vi "RT_Angle_Of_Attack_in_DLR_Navigation_Reference_System_2_v2(SubVI).vi"(8 "i":i32, 9 "V_wind [m/s]":dbl[][](array[numeric]), 10 "Rotation":T1, 11 "output cluster 2":T3) -> (3 "output cluster":T2)   [LabVIEW 2017]
uses:
  <vilib>/Analysis/_algsub.llb/Vector Norm Type.ctl
  <vilib>/Analysis/_algsub.llb/Real Vector Norm.vi
  <vilib>/Analysis/coordinate.llb/Euler Rotation Order.ctl
  <vilib>/Analysis/NI_AALPro.lvlib
panel:
  out "Elevation [deg]":dbl
  out "Azimuth [deg]":dbl
  out "AoA_yaw (deg)":dbl
  out "AoA_pitch (deg)":dbl
  out "appended array":dbl[](array[numeric])
  out "Speed_quat":dbl[](array[numeric])
  out "pitch_stream (rad)":dbl
  out "yaw_stream (rad)":dbl
  out "AoA_yaw (rad)":dbl
  out "AoA_pitch (rad)":dbl
  out "VV":dbl[](array[numeric])
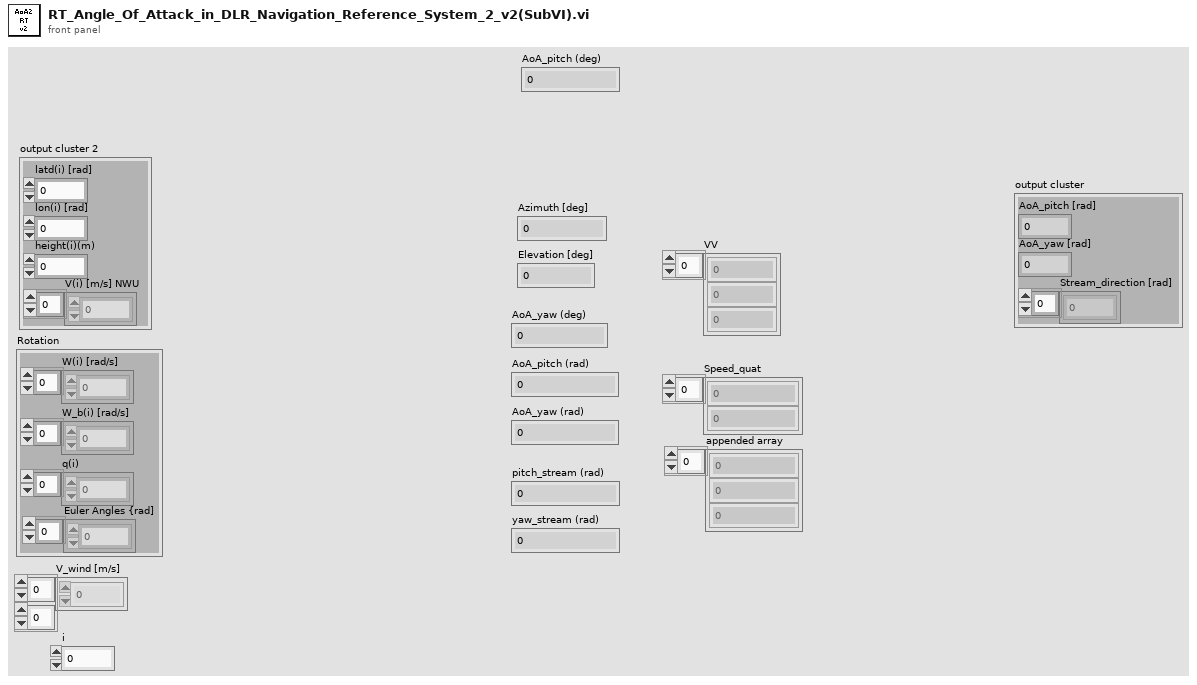
[diagram p1: front panel]
types:
  T1 = cluster{"W(i) [rad/s]":dbl[], "W_b(i) [rad/s]":dbl[], "q(i)":dbl[], "Euler Angles {rad]":dbl[]}
  T2 = cluster{"AoA_pitch [rad]":dbl, "AoA_yaw [rad]":dbl, "Stream_direction [rad]":dbl[]}
  T3 = cluster{"latd(i) [rad]":dbl, "lon(i) [rad]":dbl, "height(i)(m)":dbl, "V(i) [m/s] NWU":dbl[]}
  T4 = typedef "NI_AALPro.lvlib/Vector Norm Type.ctl" = u16
  T5 = typedef "NI_AALPro.lvlib/Euler Rotation Order.ctl" = u16
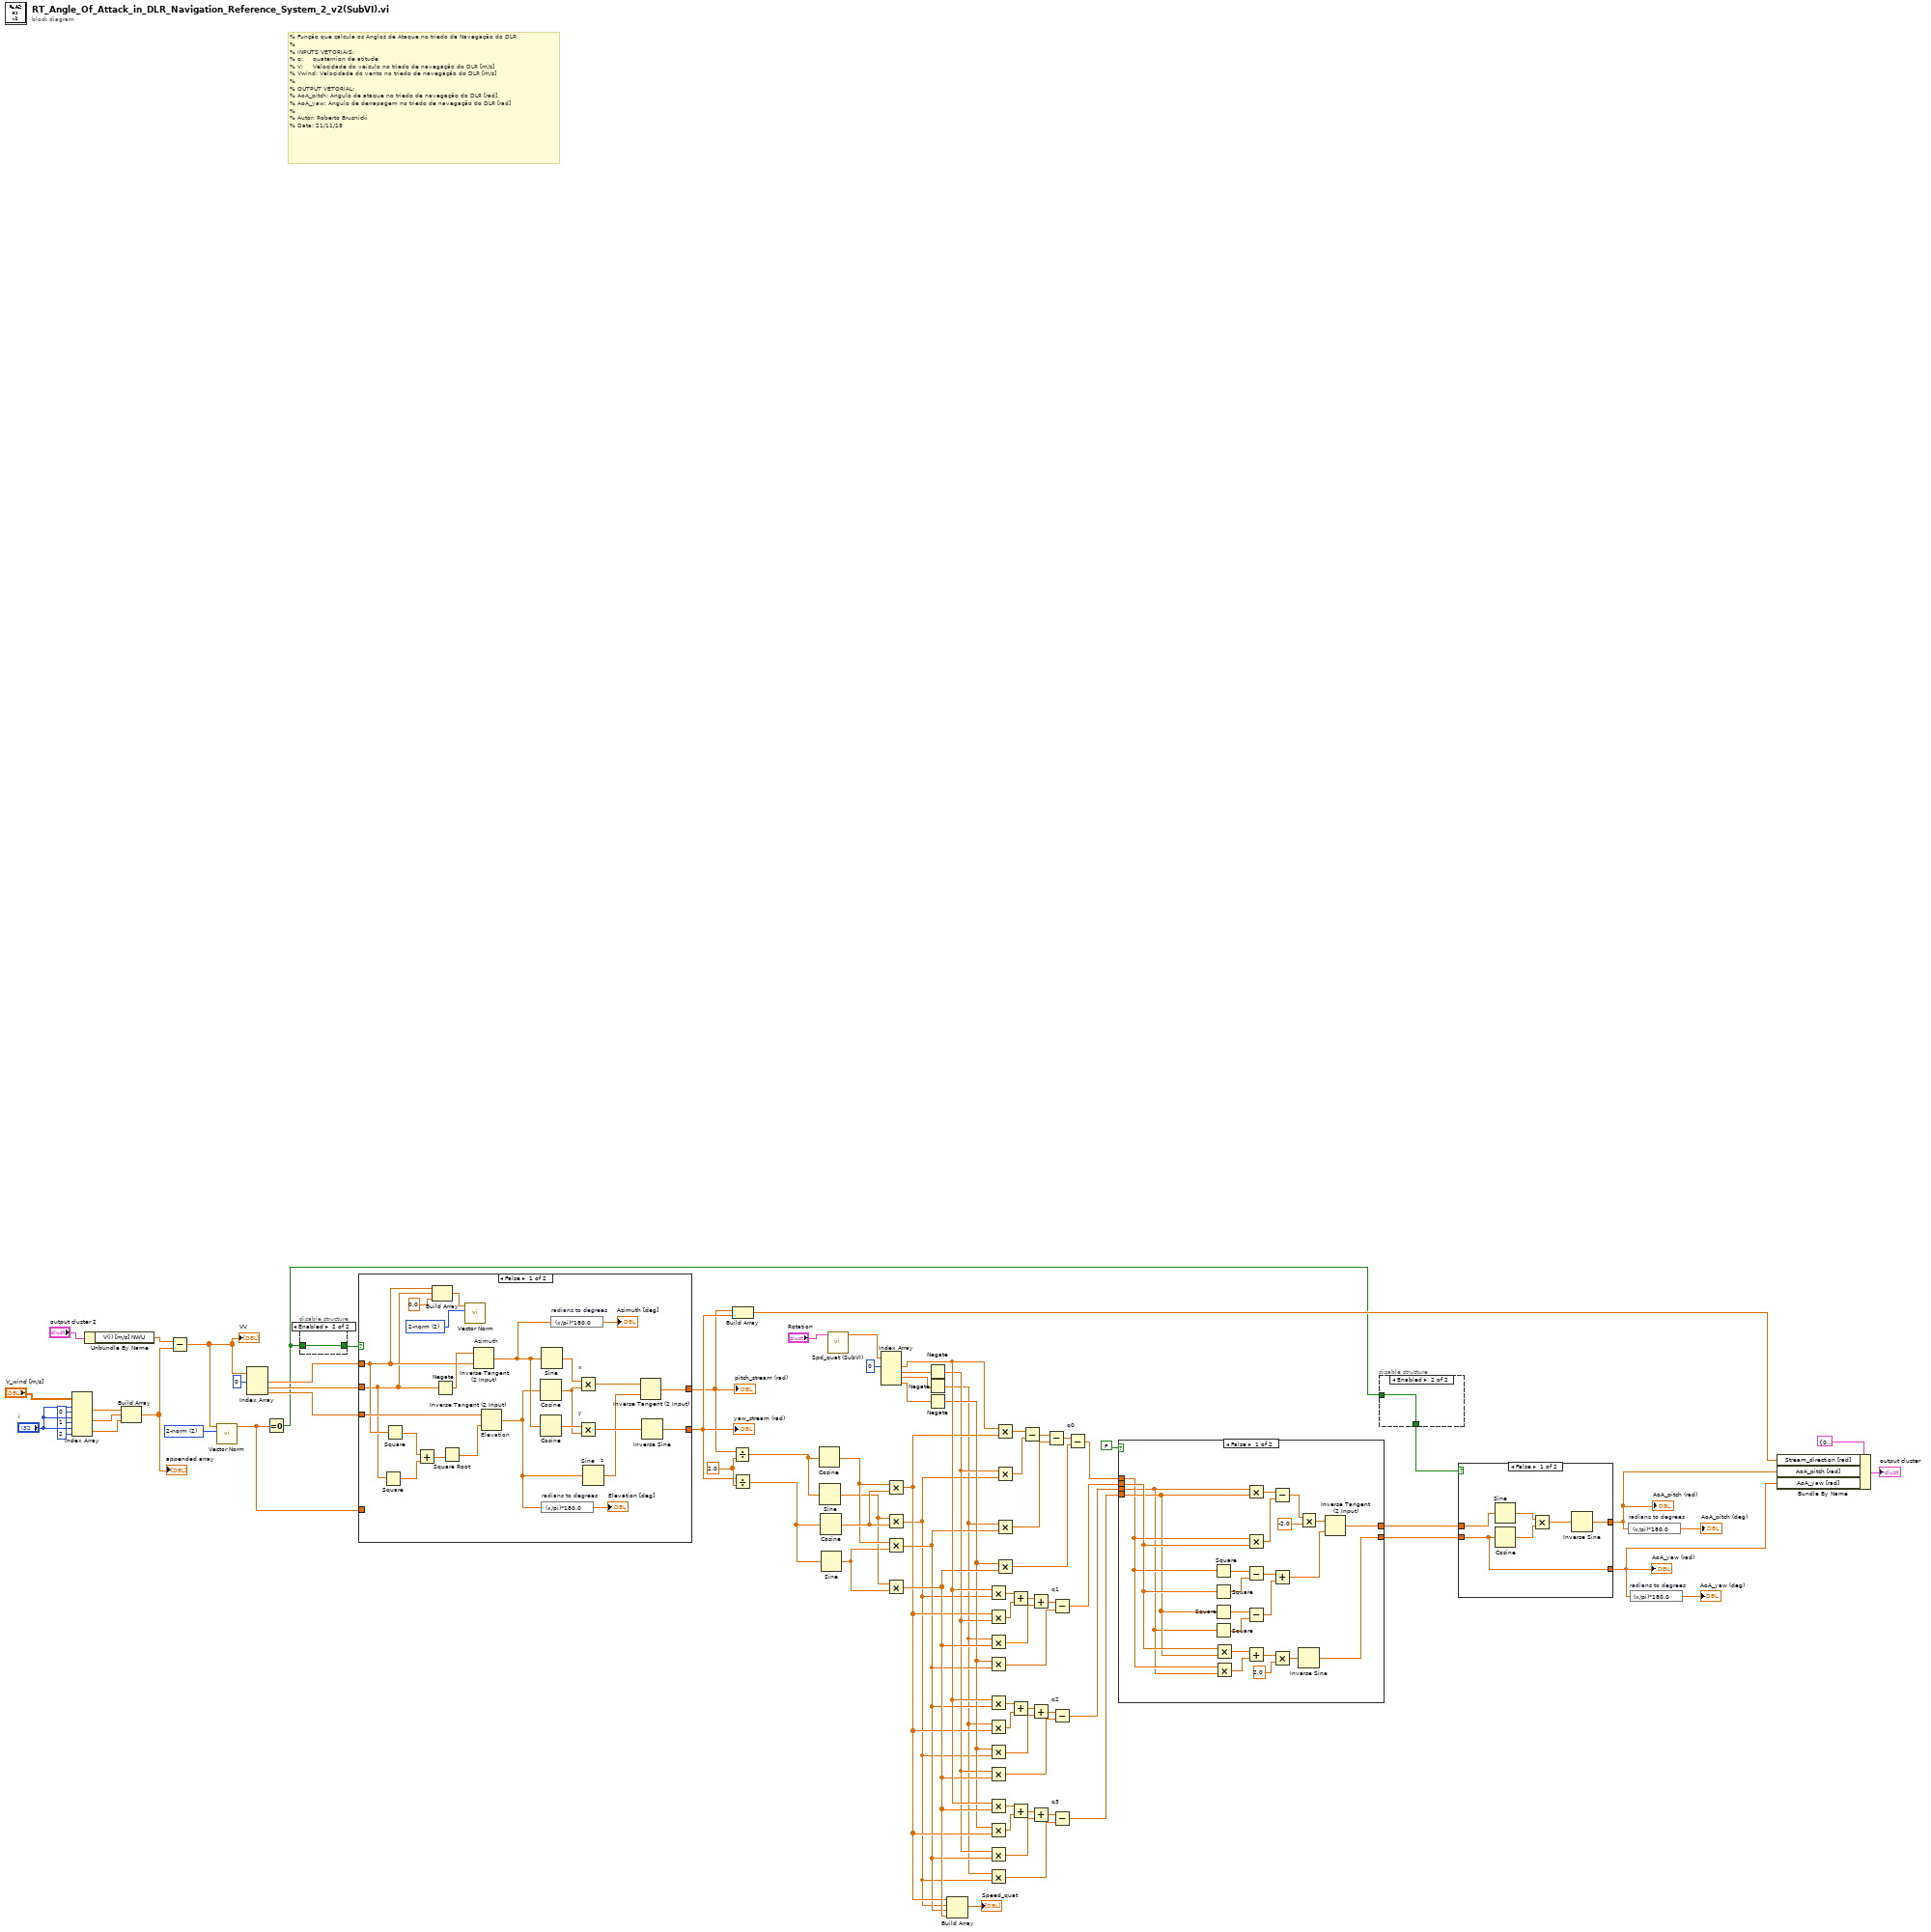
[diagram p0: block diagram]
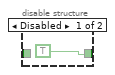
[diagram p2: hidden frame]
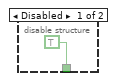
[diagram p3: hidden frame]
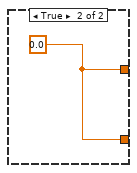
[diagram p4: hidden frame]
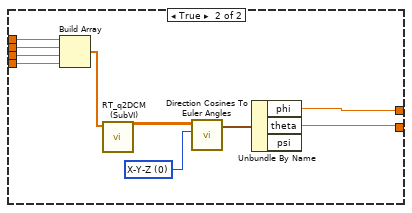
[diagram p5: hidden frame]
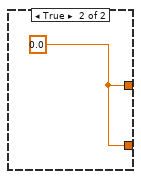
[diagram p6: hidden frame]
diagram:
  w68 = 2.0 ("y")
  w74 = T4 2 items=["1-norm"=1, "2-norm"=2, "Inf-norm"=3, "-Inf-norm"=4, "User Defined"=5] ("norm type")
  # "% Função que calcula os Anglos de Ataque no triedo de Navegação do DLR \n%\n% INPUTS VETORIAIS: \n% q:     quaternion de atitude   \n% V:     Velocidade do veículo no triedo de navegação do DLR [m/s]\n% Vwind: Velocidade do vento no triedo de navegação do DLR [m/s]\n%\n% OUTPUT VETORIAL:\n% AoA_pitch: Angulo de ataque no triedo de navegação do DLR [rad]\n% AoA_yaw: Angulo de derrapagem no triedo de navegação do DLR [rad]\n%\n% Autor: Roberto Brusnicki\n% Data: 21/11/18"
  n1 = Index Array(array="V_wind [m/s]", index (row) #1="i", index (col) #1=0 ("disabled index (col)"), index (row) #2="i", index (col) #2=1 ("disabled index (col)"), index (row) #3="i", index (col) #3=2 ("disabled index (col)")) -> (element #1=w78:dbl, element #2=w77:dbl, element #3=w76:dbl)
  n2 = Unbundle By Name("output cluster 2") -> ("V(i) [m/s] NWU"=w1:dbl[])
  n3 = Build Array(w78, w77, w76) -> (w75:dbl[])
  "appended array" <- w75
  n4 = Subtract(x=w1, y=w75) -> (x-y=w73:dbl[])
  "VV" <- w73
  n5 = call-poly <vilib>:"Vector Norm.vi"("norm type"=w74, "Input Vector"=w73) -> ("norm"=w70:dbl)  [unwired: 8 in, 1 out]
  n6 = Index Array(array=w73, index #1=0 ("index (row)")) -> (element #1=w72:dbl, element #2=w71:dbl, element #3=w17:dbl)  [unwired: 2 in]
  n7 = Equal To 0?(x=w70) -> (x = 0?=w2:bool)
  n8 = disable-structure shown="Enabled" {
    disable-tunnel: [TRUE w85] -> w3
    disable-tunnel: w2 -> [_ w85]
    frame Disabled {
    }
    frame Enabled {
    }
  }
  n9 = case shown="False" w3 {
    tunnel: [w99 w109] -> w67
    tunnel: [w96 w109] -> w66
    tunnel: w72 -> [w89 _]
    tunnel: w71 -> [w88 _]
    tunnel: w70 -> [_ _]
    tunnel: w17 -> [w107 _]
    frame False {
      w106 = T4 2 items=["1-norm"=1, "2-norm"=2, "Inf-norm"=3, "-Inf-norm"=4, "User Defined"=5] ("norm type")
      n10 = Square(x=w88) -> (x^2=w91:dbl)
      n11 = Square(x=w89) -> (x^2=w90:dbl)
      n12 = Add(x=w90, y=w91) -> (x+y=w87:dbl)
      n13 = Build Array(w89, w88, 0.0 ("element")) -> (w104:dbl[])
      n14 = Negate(x=w88) -> (-x=w108:dbl)
      n15 = Square Root(x=w87) -> (sqrt(x)=w86:dbl)
      n16 = call-poly <vilib>:"Vector Norm.vi"("norm type"=w106, "Input Vector"=w104) -> ()  [unwired: 8 in, 2 out]
      n17 = Inverse Tangent (2 Input) "Azimuth"(1:w89, 2:w108) -> (0:w95:dbl)
      n18 = Inverse Tangent (2 Input) "Elevation"(1:w86, 2:w107) -> (0:w92:dbl)
      n19 = Cosine(x=w92) -> (cos(x)=w101:dbl)
      n20 = Cosine(x=w95) -> (cos(x)=w102:dbl)
      n21 = Sine(x=w95) -> (sin(x)=w103:dbl)
      n22 = expression code="(x/pi)*180.0" "radians to degrees"(w92) -> (→"Elevation [deg]":dbl)
      n23 = expression code="(x/pi)*180.0" "radians to degrees"(w95) -> (→"Azimuth [deg]":dbl)
      n24 = Multiply "x"(x=w103, y=w101) -> (x*y=w98:dbl)
      n25 = Multiply "y"(x=w102, y=w101) -> (x*y=w100:dbl)
      n26 = Sine "z"(x=w92) -> (sin(x)=w97:dbl)
      n27 = Inverse Tangent (2 Input)(1:w97, 2:w98) -> (0:w96:dbl)
      n28 = Inverse Sine(1:w100) -> (0:w99:dbl)
    }
    frame True {
      w109 = 0.0 ("Speed_pitch (rad)")
    }
  }
  "pitch_stream (rad)" <- w66
  "yaw_stream (rad)" <- w67
  n29 = Divide(x=w66, y=w68) -> (x/y=w65:dbl)
  n30 = Build Array(w66, w67) -> (w9:dbl[])
  n31 = Divide(x=w67, y=w68) -> (x/y=w64:dbl)
  n32 = Cosine(x=w65) -> (cos(x)=w62:dbl)
  n33 = Sine(x=w65) -> (sin(x)=w61:dbl)
  n34 = Cosine(x=w64) -> (cos(x)=w63:dbl)
  n35 = Sine(x=w64) -> (sin(x)=w60:dbl)
  n36 = call "Spd_quat (SubVI).vi"("Rotation"="Rotation") -> ("Array"=w13:dbl[])  [unwired: 10 in]
  n37 = Index Array(array=w13, index #1=0 ("index")) -> (element #1=w31:dbl, element #2=w56:dbl, element #3=w57:dbl, element #4=w58:dbl)  [unwired: 3 in]
  n38 = Multiply(x=w62, y=w63) -> (x*y=w28:dbl)
  n39 = Multiply(x=w61, y=w63) -> (x*y=w24:dbl)
  n40 = Multiply(x=w62, y=w60) -> (x*y=w26:dbl)
  n41 = Multiply(x=w61, y=w60) -> (x*y=w30:dbl)
  n42 = Negate(x=w56) -> (-x=w27:dbl)
  n43 = Negate(x=w57) -> (-x=w25:dbl)
  n44 = Negate(x=w58) -> (-x=w29:dbl)
  n45 = Build Array(w28, w24, w26, w30) -> (→"Speed_quat":dbl[])
  n46 = Multiply(x=w31, y=w24) -> (x*y=w49:dbl)
  n47 = Multiply(x=w28, y=w27) -> (x*y=w48:dbl)
  n48 = Multiply(x=w25, y=w30) -> (x*y=w45:dbl)
  n49 = Multiply(x=w29, y=w26) -> (x*y=w44:dbl)
  n50 = Multiply(x=w31, y=w26) -> (x*y=w38:dbl)
  n51 = Multiply(x=w25, y=w28) -> (x*y=w39:dbl)
  n52 = Multiply(x=w29, y=w24) -> (x*y=w42:dbl)
  n53 = Multiply(x=w27, y=w30) -> (x*y=w43:dbl)
  n54 = Multiply(x=w31, y=w30) -> (x*y=w37:dbl)
  n55 = Multiply(x=w29, y=w28) -> (x*y=w36:dbl)
  n56 = Multiply(x=w27, y=w26) -> (x*y=w33:dbl)
  n57 = Multiply(x=w25, y=w24) -> (x*y=w32:dbl)
  n58 = Multiply(x=w31, y=w28) -> (x*y=w55:dbl)
  n59 = Multiply(x=w27, y=w24) -> (x*y=w54:dbl)
  n60 = Multiply(x=w25, y=w26) -> (x*y=w52:dbl)
  n61 = Multiply(x=w29, y=w30) -> (x*y=w50:dbl)
  n62 = Add(x=w49, y=w48) -> (x+y=w47:dbl)
  n63 = Add(x=w38, y=w39) -> (x+y=w40:dbl)
  n64 = Add(x=w37, y=w36) -> (x+y=w35:dbl)
  n65 = Subtract(x=w55, y=w54) -> (x-y=w53:dbl)
  n66 = Add(x=w47, y=w45) -> (x+y=w46:dbl)
  n67 = Add(x=w40, y=w42) -> (x+y=w41:dbl)
  n68 = Add(x=w35, y=w33) -> (x+y=w34:dbl)
  n69 = Subtract(x=w53, y=w52) -> (x-y=w51:dbl)
  n70 = Subtract "q1"(x=w46, y=w44) -> (x-y=w22:dbl)
  n71 = Subtract "q2"(x=w41, y=w43) -> (x-y=w21:dbl)
  n72 = Subtract "q3"(x=w34, y=w32) -> (x-y=w20:dbl)
  n73 = Subtract "q0"(x=w51, y=w50) -> (x-y=w23:dbl)
  n74 = case shown="False" FALSE {
    tunnel: w23 -> [w117 w142]
    tunnel: w22 -> [w119 w141]
    tunnel: w21 -> [w116 w140]
    tunnel: w20 -> [w118 w139]
    tunnel: [w120 w137] -> w19
    tunnel: [w110 w136] -> w18
    frame False {
      n75 = Square(x=w117) -> (x^2=w127:dbl)
      n76 = Square(x=w119) -> (x^2=w126:dbl)
      n77 = Square(x=w118) -> (x^2=w125:dbl)
      n78 = Square(x=w116) -> (x^2=w124:dbl)
      n79 = Multiply(x=w119, y=w118) -> (x*y=w115:dbl)
      n80 = Multiply(x=w117, y=w116) -> (x*y=w114:dbl)
      n81 = Multiply(x=w116, y=w118) -> (x*y=w132:dbl)
      n82 = Multiply(x=w117, y=w119) -> (x*y=w131:dbl)
      n83 = Subtract(x=w127, y=w126) -> (x-y=w123:dbl)
      n84 = Subtract(x=w125, y=w124) -> (x-y=w122:dbl)
      n85 = Add(x=w115, y=w114) -> (x+y=w112:dbl)
      n86 = Subtract(x=w132, y=w131) -> (x-y=w130:dbl)
      n87 = Add(x=w123, y=w122) -> (x+y=w121:dbl)
      n88 = Multiply(x=w112, y=2.0) -> (x*y=w111:dbl)
      n89 = Multiply(x=w130, y=-2.0) -> (x*y=w128:dbl)
      n90 = Inverse Sine(1:w111) -> (0:w110:dbl)
      n91 = Inverse Tangent (2 Input)(1:w121, 2:w128) -> (0:w120:dbl)
    }
    frame True {
      w134 = T5 0 items=["X-Y-Z", "X-Z-Y", "Y-X-Z", "Y-Z-X", "Z-X-Y", "Z-Y-X", "X-Y-X", "X-Z-X", "Y-X-Y", "Y-Z-Y", "Z-X-Z", "Z-Y-Z"] ("rotation order")
      n92 = Build Array(w142, w141, w140, w139) -> (w138:dbl[])
      n93 = call "RT_q2DCM (SubVI).vi"("Quaternion"=w138) -> ("DCM"=w135:dbl[][])  [unwired: 10 in]
      n94 = call <vilib>:"Direction Cosines To Euler Angles.vi"("rotation order"=w134, "Direction Cosines"=w135) -> ("Euler Angles"=w133:cluster{"phi":dbl, "theta":dbl, "psi":dbl})  [unwired: 8 in, 1 out]
      n95 = Unbundle By Name(w133) -> ("phi"=w137:dbl, "theta"=w136:dbl)  [unwired: 1 out]
    }
  }
  n96 = disable-structure shown="Enabled" {
    disable-tunnel: w2 -> [_ w144]
    disable-tunnel: [TRUE ("x = 0?") w144] -> w5
    frame Disabled {
    }
    frame Enabled {
    }
  }
  n97 = case shown="False" w5 {
    tunnel: w19 -> [w150 _]
    tunnel: [w146 w151] -> w11
    tunnel: w18 -> [w145 _]
    tunnel: [w145 w151] -> w10
    frame False {
      n98 = Sine(x=w150) -> (sin(x)=w149:dbl)
      n99 = Cosine(x=w145) -> (cos(x)=w148:dbl)
      n100 = Multiply(x=w149, y=w148) -> (x*y=w147:dbl)
      n101 = Inverse Sine(1:w147) -> (0:w146:dbl)
    }
    frame True {
      w151 = 0.0
    }
  }
  "AoA_pitch (rad)" <- w11
  "AoA_yaw (rad)" <- w10
  n102 = expression code="(x/pi)*180.0" "radians to degrees"(w11) -> (→"AoA_pitch (deg)":dbl)
  n103 = expression code="(x/pi)*180.0" "radians to degrees"(w10) -> (→"AoA_yaw (deg)":dbl)
  n104 = Bundle By Name(cluster=T2 {"AoA_pitch [rad]"=0.0, "AoA_yaw [rad]"=0.0, "Stream_direction [rad]"=[]} ("output cluster 4"), "Stream_direction [rad]"=w9, "AoA_pitch [rad]"=w11, "AoA_yaw [rad]"=w10) -> (→"output cluster":T2)
